vi "Simple TCP - Client - Copy - Copy.vi"() -> ()   [LabVIEW 2021]
doc: "Demonstrates how to open a connection to an TCP server, read the data being sent, and display the data on a chart. This VI is designed to stop if the TCP connection is terminated."
uses:
  <vilib>/Analysis/3filter.llb/Butterworth Filter (DBL).vi
  <vilib>/Analysis/NI_AALBase.lvlib
  <vilib>/ptbypt/NI_PtbyPt.lvlib
panel:
  out "Filtered":dbl[](graph)
  out "Array Size 3":u32
  out "Delayed RMS2>RMS1 for 3 data":dynamicdata(graph)
  out "RMS2>RMS1 for 3 data":dynamicdata(graph)
  out "Array Size":u32
  out "RMS2>RMS1":dynamicdata(graph)
  out "RMS1":dynamicdata(graph)
  out "RMS2":dynamicdata(graph)
  out "Raw Data Collected":dynamicdata(graph)
  in  "Boolean":bool
  in  "Server Closed":string="The server VI closed the connection."
  out "Raw Data":dbl[](graph)
  in  "Stop":bool
  # "Overview: Demonstrates the use of the TCP functions to connect to a TCP server VI and receive data.\nInstructions:\n1. Ensure Simple TCP - Server.vi is already running.\n2. Run the VI.\n3. Click Stop to stop the VI. Note that if you stop the server VI, this VI will stop automatically."
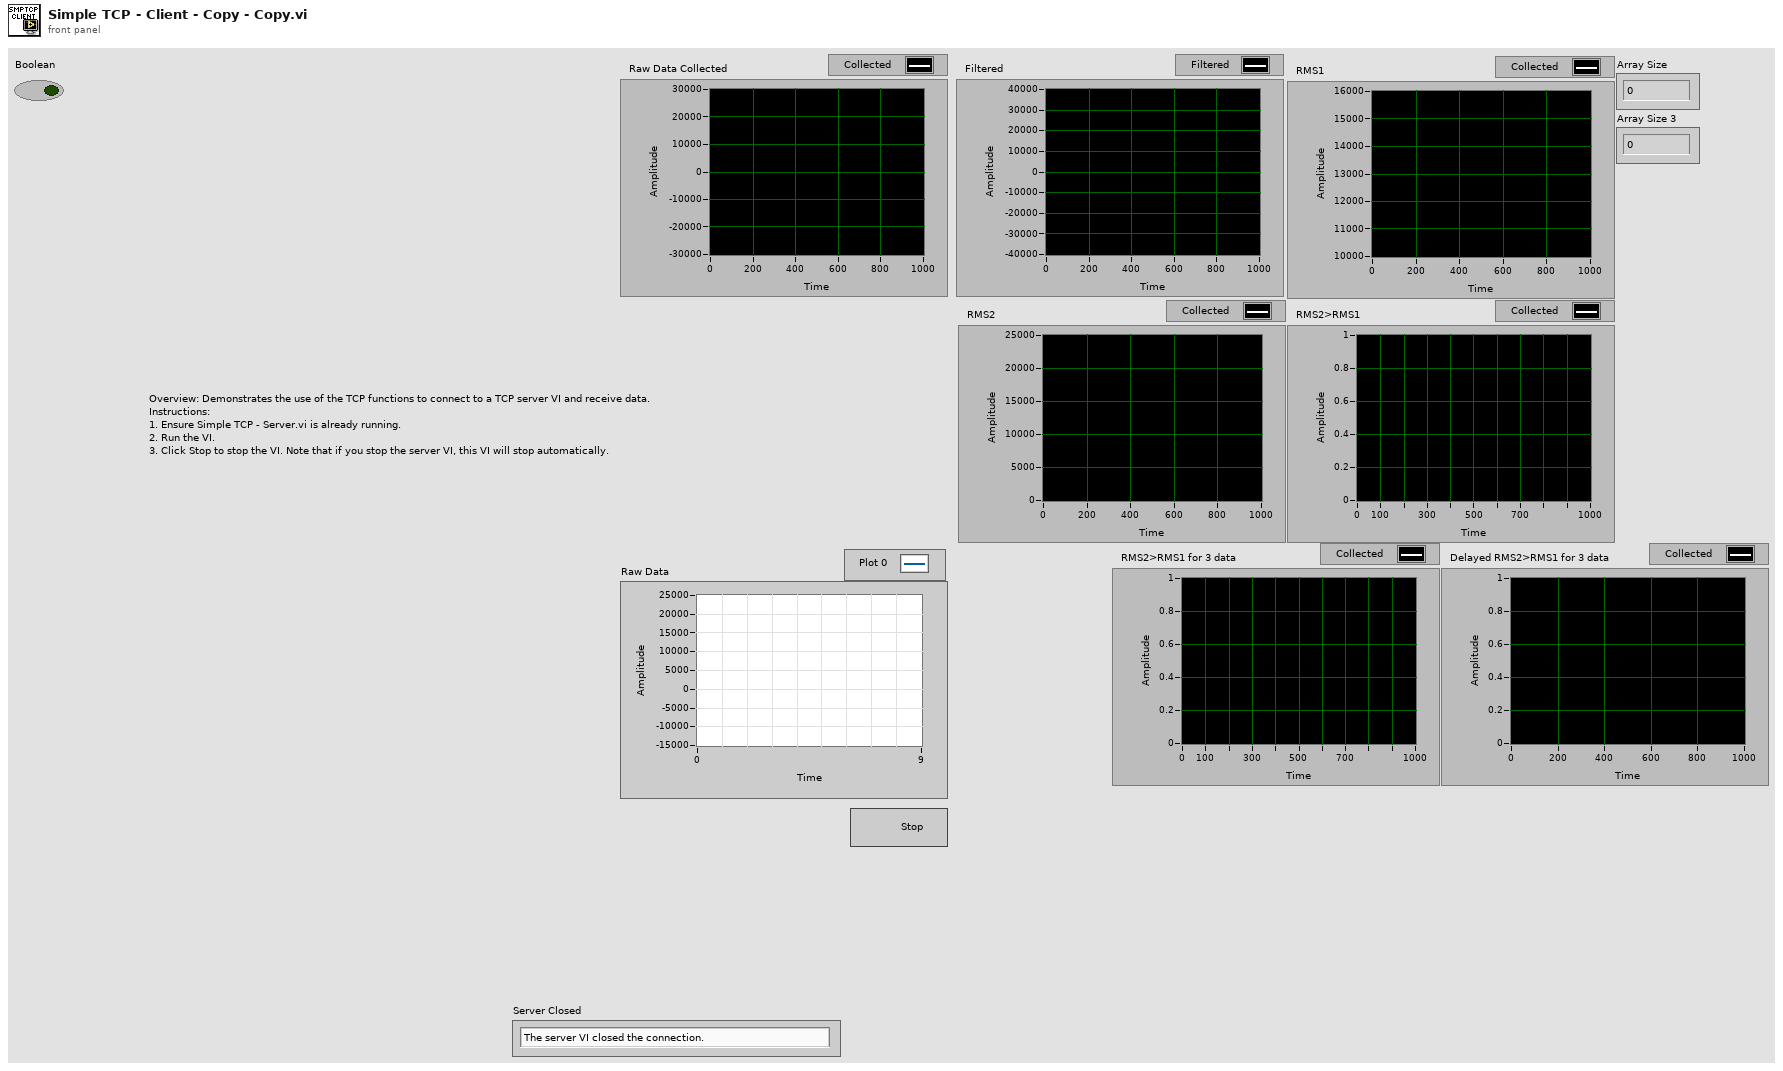
[diagram p1: front panel]
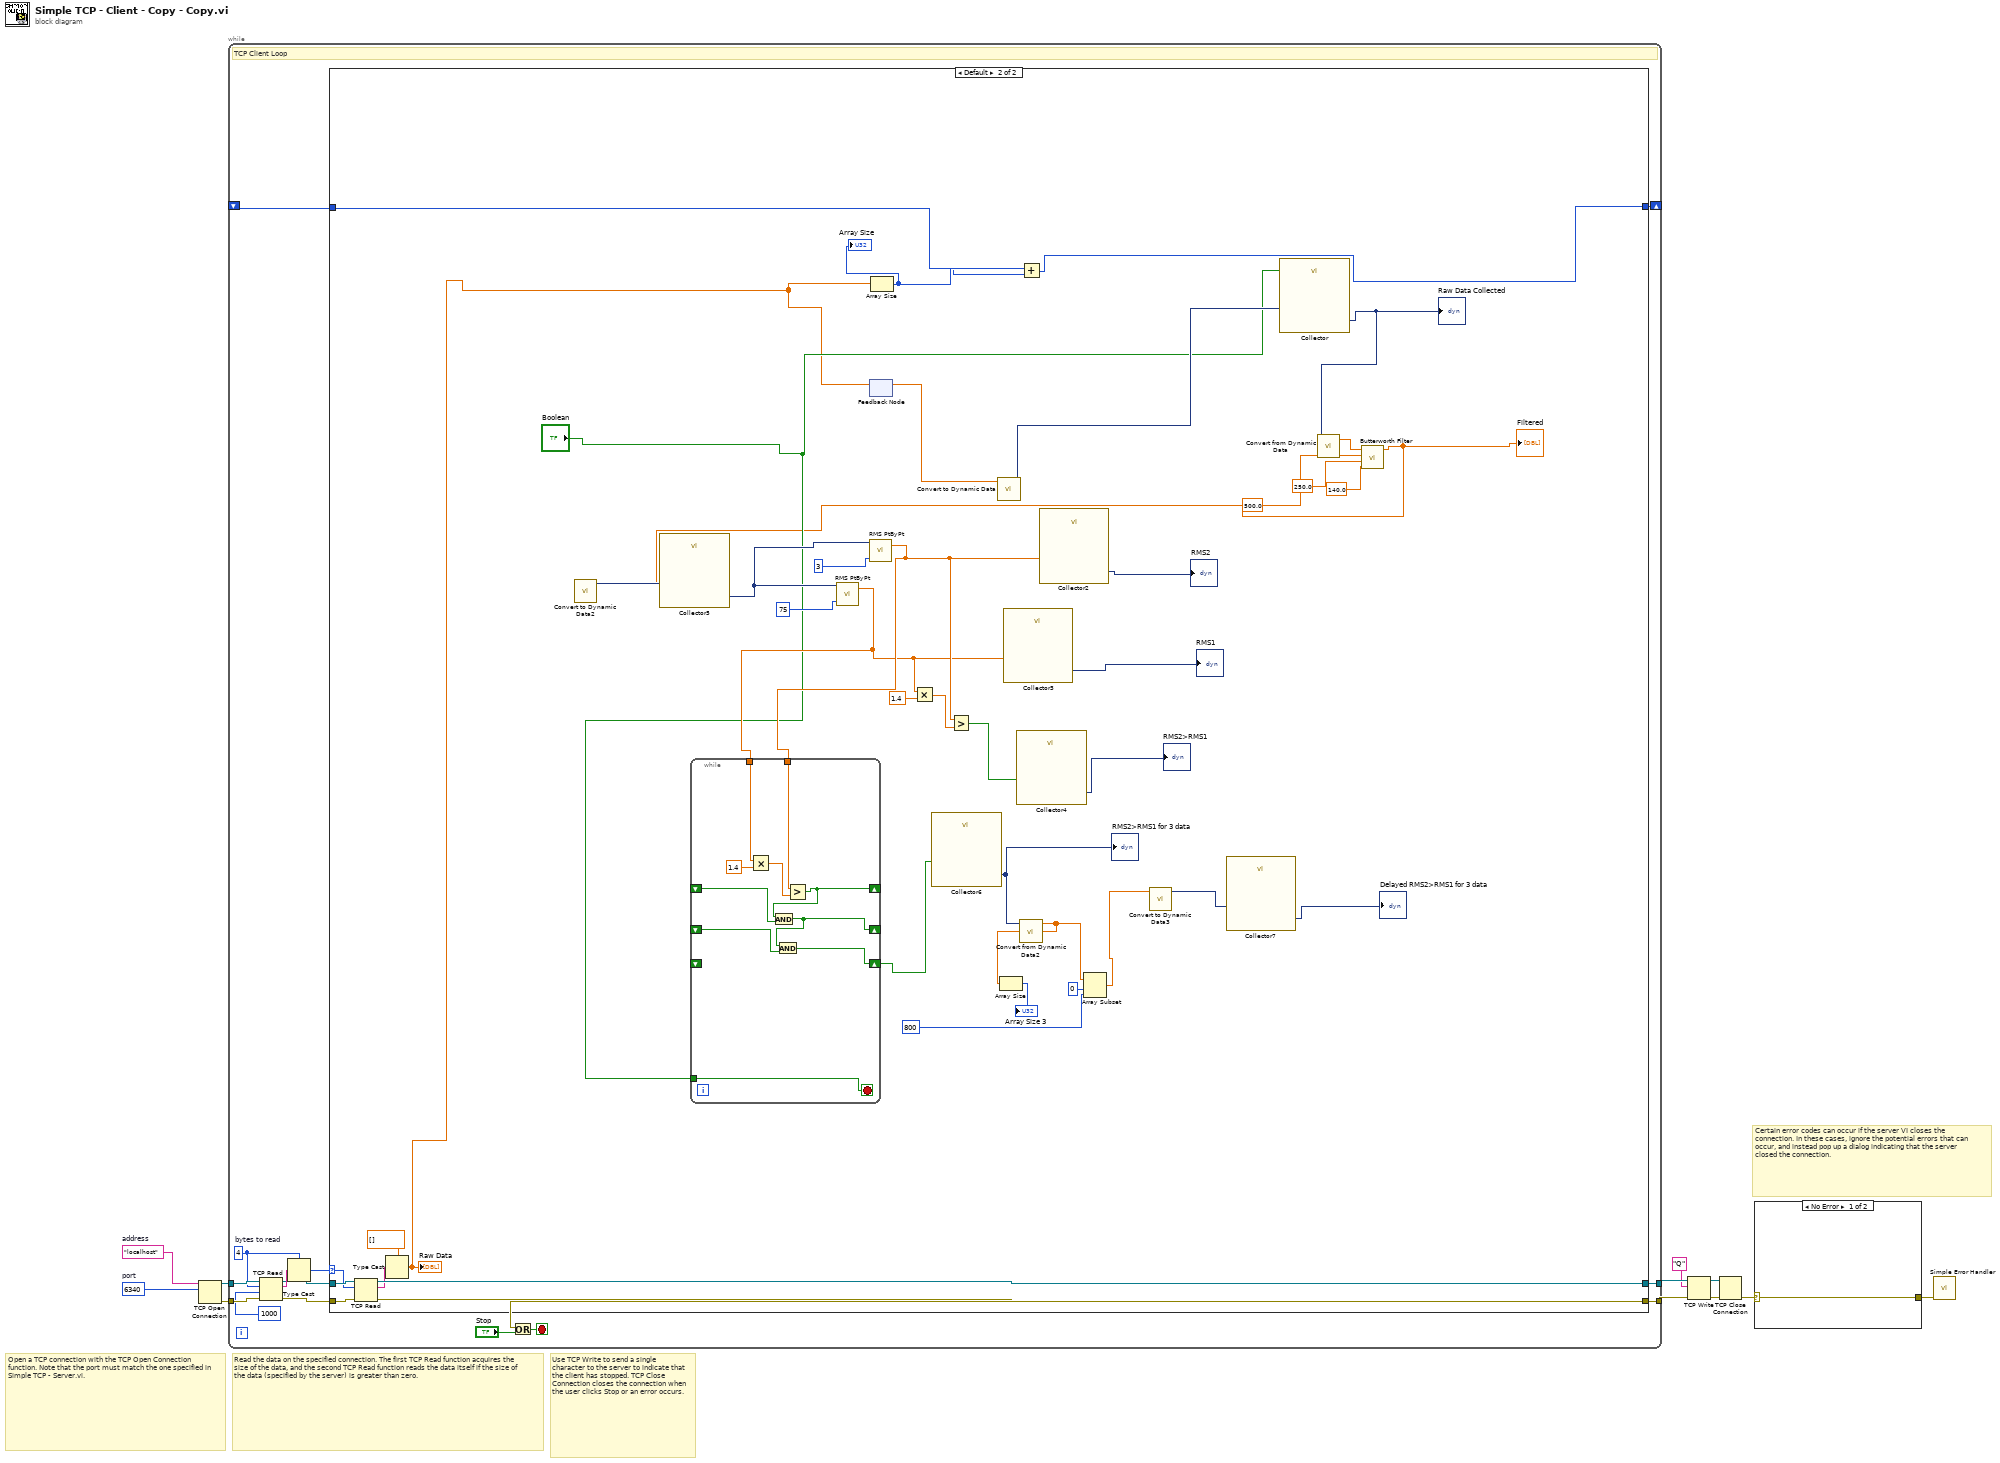
[diagram p0: block diagram]
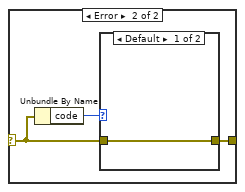
[diagram p2: hidden frame]
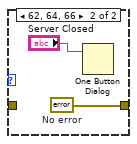
[diagram p3: hidden frame]
diagram:
  w1 = u16 6340  # port
  w2 = "localhost"  # address
  # "Certain error codes can occur if the server VI closes the connection. In these cases, ignore the potential errors that can occur, and instead pop up a dialog indicating that the server closed the connection."
  # "Use TCP Write to send a single character to the server to indicate that the client has stopped. TCP Close Connection closes the connection when the user clicks Stop or an error occurs."
  # "Read the data on the specified connection. The first TCP Read function acquires the size of the data, and the second TCP Read function reads the data itself if the size of the data (specified by the server) is greater than zero."
  # "Open a TCP connection with the TCP Open Connection function. Note that the port must match the one specified in Simple TCP - Server.vi."
  n1 = TCP Open Connection(address=w2, remote port or service name=w1) -> (connection ID=w11:refnum<k5>, error out=w10:errorcluster)  [unwired: 3 in]
  n2 = while {
    tunnel: w10 -> [w21]
    tunnel: w11 -> [w22]
    tunnel: [w17] -> w8
    tunnel: [w16] -> w6
    shift-right: [w12] -> _
    shift-left: _ -> [w13]
    stop <- w18 stop-if-true
    w20 = 4  # bytes to read
    # "TCP Client Loop"
    n3 = TCP Read(connection ID=w22, bytes to read=w20, error in (no error)=w21, 9:1000 ("timeout ms (25000)")) -> (connection ID out=w24:refnum<k5>, data out=w25:string, error out=w23:errorcluster)  [unwired: 1 in]
    n4 = Type Cast(type=w20, x=w25) -> (*(type *) &x=w15:i32)
    n5 = case shown="Default" w15 {
      selector: w15 -> [_ w63]
      tunnel: w24 -> [w28 w69]
      tunnel: w23 -> [w27 w68]
      tunnel: [w28 w66] -> w17
      tunnel: [w27 w65] -> w16
      tunnel: w13 -> [w26 w32]
      tunnel: [w26 w31] -> w12
      frame ..0 {
        # "The server has not written any data"
      }
      frame Default {
        n6 = TCP Read(connection ID=w69, bytes to read=w63, error in (no error)=w68) -> (connection ID out=w66:refnum<k5>, data out=w64:string, error out=w65:errorcluster)  [unwired: 2 in]
        n7 = Type Cast(type=dbl[] [] ("chart"), x=w64) -> (*(type *) &x=w30:dbl[])
        "Raw Data" <- w30
        n8 = feedback #1() -> (w46:dbl[])  [unwired: 1 in]
        n9 = feedback-in #1(w30) -> ()
        n10 = Array Size(array=w30) -> (size(s)=w45:i32)
        "Array Size" <- w45
        n11 = call "Convert to Dynamic Data"("Array"=w46) -> ("Dynamic Data Type"=w55:dynamicdata)  [unwired: 3 in]
        n12 = Add(x=w45, y=w32) -> (x+y=w31:i32)
        n13 = call "Collector"("Enable"="Boolean", "Signals"=w55) -> ("Collected Signals"=w58:dynamicdata)  [unwired: 8 in, 1 out]
        "Raw Data Collected" <- w58
        n14 = call "Convert from Dynamic Data"("Dynamic Data Type"=w58) -> ("Array"=w59:dbl[])  [unwired: 3 in]
        n15 = call-poly <vilib>:"Butterworth Filter.vi"("low cutoff freq: fl"=140.0, "high cutoff freq: fh"=250.0, "sampling freq: fs"=500.0, "X"=w59) -> ("Filtered X"=w29:dbl[])  [unwired: 4 in, 1 out]
        "Filtered" <- w29
        n16 = call "Convert to Dynamic Data2"("Array"=w29) -> ("Dynamic Data Type"=w48:dynamicdata)  [unwired: 3 in]
        n17 = call "Collector5"("Signals"=w48) -> ("Collected Signals"=w47:dynamicdata)  [unwired: 9 in, 1 out]
        n18 = call <vilib>:"RMS PtByPt.vi"("sample length"=75, "x"=w47) -> ("rms value"=w43:dbl)  [unwired: 2 in, 1 out]
        n19 = call <vilib>:"RMS PtByPt.vi"("sample length"=3, "x"=w47) -> ("rms value"=w44:dbl)  [unwired: 2 in, 1 out]
        n20 = while {
          tunnel: w44 -> [w77]
          tunnel: w43 -> [w76]
          shift-right: [w71] -> _
          shift-left: _ -> [w72]
          shift-right: [w74] -> _
          shift-left: _ -> [w73]
          tunnel: "Boolean" -> [w75]
          shift-right: [w70] -> w40
          shift-left: _ -> [_]
          stop <- w75 stop-if-true
          n21 = Multiply(x=w76, y=1.4) -> (x*y=w78:dbl)
          n22 = Greater?(x=w77, y=w78) -> (0:w74:bool)
          n23 = And(x=w74, y=w73) -> (x .and. y?=w71:bool)
          n24 = And(x=w71, y=w72) -> (x .and. y?=w70:bool)
        }
        n25 = Multiply(x=w43, y=1.4) -> (x*y=w51:dbl)
        n26 = call "Collector6"("Signals"=w40) -> ("Collected Signals"=w38:dynamicdata)  [unwired: 9 in, 1 out]
        "RMS2>RMS1 for 3 data" <- w38
        n27 = Greater?(x=w44, y=w51) -> (0:w50:bool)
        n28 = call "Collector3"("Signals"=w43) -> ("Collected Signals"=→"RMS1":dynamicdata)  [unwired: 9 in, 1 out]
        n29 = call "Collector4"("Signals"=w50) -> ("Collected Signals"=→"RMS2>RMS1":dynamicdata)  [unwired: 9 in, 1 out]
        n30 = call "Convert from Dynamic Data2"("Dynamic Data Type"=w38) -> ("Array"=w35:dbl[])  [unwired: 3 in]
        n31 = Array Size(array=w35) -> (size(s)=→"Array Size 3":i32)
        n32 = call "Collector2"("Signals"=w44) -> ("Collected Signals"=→"RMS2":dynamicdata)  [unwired: 9 in, 1 out]
        n33 = Array Subset(array=w35, index=0, length=800 ("index")) -> (w33:dbl[])
        n34 = call "Convert to Dynamic Data3"("Array"=w33) -> ("Dynamic Data Type"=w39:dynamicdata)  [unwired: 3 in]
        n35 = call "Collector7"("Signals"=w39) -> ("Collected Signals"=→"Delayed RMS2>RMS1 for 3 data":dynamicdata)  [unwired: 9 in, 1 out]
      }
    }
    n36 = Or(x=w16, y="Stop") -> (x .or. y?=w18:bool)
  }
  n37 = TCP Write(connection ID=w8, data in="Q", error in (no error)=w6) -> (connection ID out=w9:refnum<k5>, error out=w7:errorcluster)  [unwired: 2 out]
  n38 = TCP Close Connection(connection ID=w9, error in (no error)=w7) -> (error out=w4:errorcluster)  [unwired: 1 in, 1 out]
  n39 = case shown="No Error" w4 {
    selector: w4 -> [w80 w82]
    tunnel: [w80 w81] -> w3
    frame No Error {
    }
    frame Error {
      n40 = Unbundle By Name(w82) -> ("code"=w83:i32)
      n41 = case shown="Default" w83 {
        tunnel: w82 -> [w84 _]
        tunnel: [w84 w86] -> w81
        frame Default {
        }
        frame 62, 64, 66 {
          w86 = errorcluster {"status"=FALSE, "code"=0, "source"=""}  # No error
          n42 = One Button Dialog(message="Server Closed") -> ()  [unwired: 1 in, 1 out]
        }
      }
    }
  }
  n43 = call <vilib>:"Simple Error Handler.vi"("error in (no error)"=w3) -> ()  [unwired: 4 in, 5 out]
